vi "sq_test.vi"() -> ()   [LabVIEW 2011]
uses:
  <vilib>/Platform/TimedLoop/XDataNode/timing_clust.ctl
  <vilib>/Platform/TimedLoop/XDataNode/nitl_modes.ctl
  <vilib>/Platform/TimedLoop/XDataNode/wakeup.ctl
  <vilib>/Platform/TimedLoop/XDataNode/XDataNode.xnode
  <vilib>/Platform/TimedLoop/XDataNode/XDNodeRunTimeDep.lvlib
panel:
  in  "Num read":u8
  in  "Init sequences":T1={"Cluster"={"Cmd bytes"=[0, 99, 145], "Send"=FALSE}, "Cluster 2"={"Cmd bytes"=[0, 107, 145, 119, 255], "Send"=FALSE}, "Cluster 3"={"Cmd bytes"=[0, 103, 145, 119, 255], "Send"=FALSE}, "Cluster 4"={"Cmd bytes"=[], "Send"=FALSE}} {"Cluster 4"."Cmd bytes" format="%.0x"; "Cluster 3"."Cmd bytes" format="%.0x"; "Cluster 2"."Cmd bytes" format="%.0x"; "Cluster"."Cmd bytes" format="%.0x"}
  in  "Continuous 2":bool
  in  "Bit rate":dbl=400000.0 min=40000.0 max=2000000.0 format="%#_3p"
  in  "Address":u8=84 max=127 step=1 format="%2x"
  in  "Bus":u8 max=2 step=1
  in  "Pulse count":i16(slide) min=-2047 max=2047 scale=-1700.0..1700.0
  in  "Continuous":bool
  in  "Step":bool
  in  "Send":bool
  in  "stop":bool
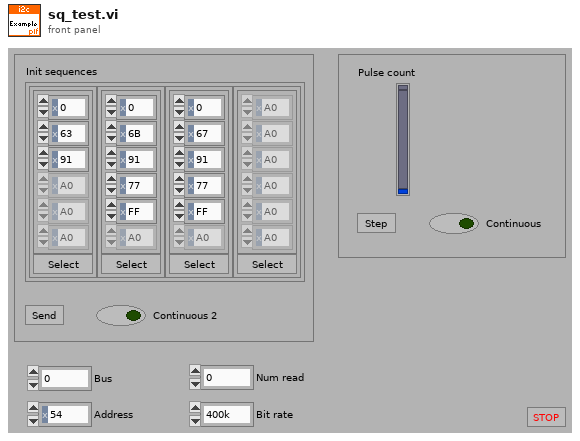
[diagram p1: front panel]
types:
  T1 = cluster{"Cluster":cluster{"Cmd bytes":u8[], "Send":bool}, "Cluster 2":cluster{"Cmd bytes":u8[], "Send":bool}, "Cluster 3":cluster{"Cmd bytes":u8[], "Send":bool}, "Cluster 4":cluster{"Cmd bytes":u8[], "Send":bool}}
  T2 = typedef "i2c_interface.ctl" = cluster{"FPGA VI Reference":T3}
  T3 = typedef "fpga_reference.ctl" = refnum<k20>
  T4 = typedef "XDNodeRunTimeDep.lvlib/timing_clust.ctl" = cluster{"Expected End [f-1]":u64, "Actual End [f-1]":u64, "Finished Late? [f-1]":bool, "Expected End [i-1]":u64, "Actual End [i-1]":u64, "Finished Late? [i-1]":bool, "Expected Start [i]":u64, "Actual Start [i]":u64, "Expected Start [f]":u64, "Actual Start [f]":u64, "Source Name":string, "Structure Name":string, "Period":i64, "Deadline":i64, "Offset":i64, "Start":i64, "Priority":i32, "Timeout":i32, "Mode":T5, "Wakeup Reason":T6, "Error":errorcluster, "Source Type":string, "Secondary Source Type":string, "Global End Time":u64, "Global Start Time":u64, "Frame Duration":u64, "Iteration Duration":u64, "Assigned CPU":i32, "I/O Scan Engine Mode":u32}
  T5 = typedef "XDNodeRunTimeDep.lvlib/nitl_modes.ctl" = enum32{"No Change", "Process missed periods, maintain original phase", "Discard missed periods, maintain original phase", "Process missed periods, ignore original phase", "Discard missed periods, ignore original phase"}
  T6 = typedef "XDNodeRunTimeDep.lvlib/wakeup.ctl" = enum32{"Normal", "Aborted", "Asynchronous wakeup", "Timing source error", "Timed loop error", "Timeout"}
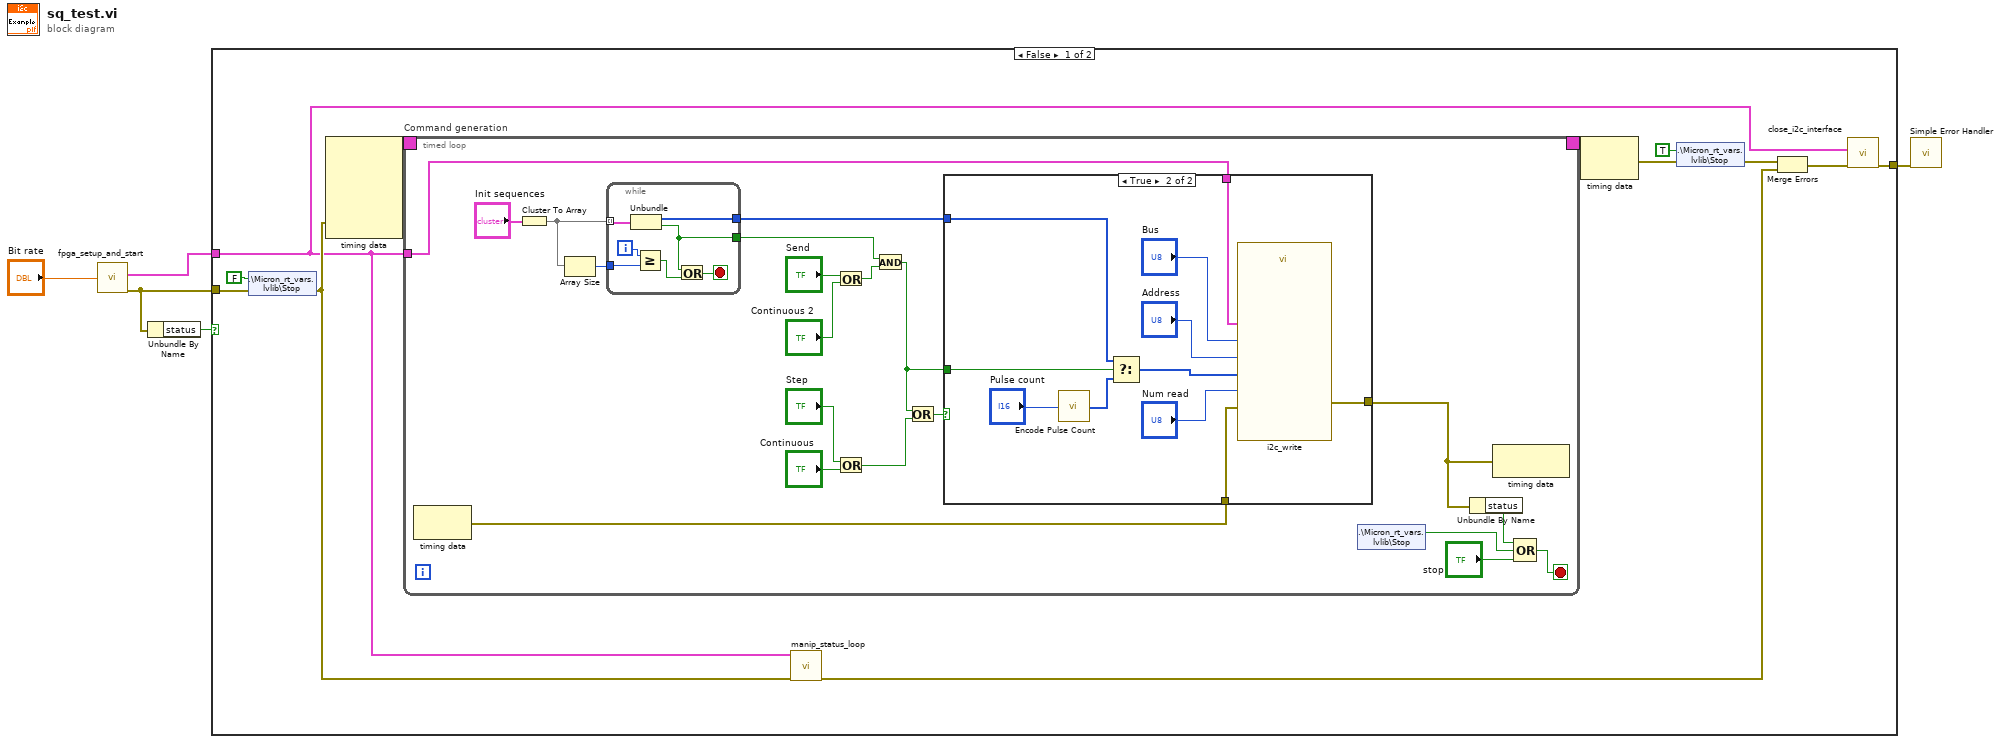
[diagram p0: block diagram]
diagram:
  n1 = call "fpga_setup_and_start.vi"("Bit rate"="Bit rate") -> ("error out"=w3:errorcluster, "I2C interface"=w2:T2)  [unwired: 9 in]
  n2 = Unbundle By Name(w3) -> ("status"=w1:bool)
  n3 = case shown="False" w1 {
    tunnel: [w15 w67] -> w5
    tunnel: w3 -> [w7 w67]
    tunnel: w2 -> [w6 _]
    frame False {
      n4 = shared-variable ".\\Micron_rt_vars.lvlib\\Stop"(FALSE ("Stop"), error in=w7) -> (error out=w8:errorcluster)
      n5 = node-c288(w8) -> (w17:T4)  [unwired: 4 in]
      n6 = timed-loop "Command generation" {
        timing: w17 -> [_]
        timing-out: [_] -> w16
        tunnel: w6 -> [w31]
        stop <- w36 stop-if-true
        n7 = node-c288() -> (w30:errorcluster)  [unwired: 1 in]
        n8 = Cluster To Array(cluster="Init sequences") -> (array=w23:cluster{"Cmd bytes":u8[], "Send":bool}[])
        n9 = Array Size(array=w23) -> (size(s)=w22:i32)
        n10 = while {
          tunnel: w23 -> [w44] mode=indexing
          tunnel: [w43] -> w21
          tunnel: w22 -> [w41]
          tunnel: [w38] -> w19
          i -> [w40]
          stop <- w42 stop-if-true
          n11 = Unbundle(w44) -> ("Cmd bytes"=w43:u8[], "Send"=w38:bool)
          n12 = Greater Or Equal?(x=w40, y=w41) -> (x >= y?=w39:bool)
          n13 = Or(x=w38, y=w39) -> (x .or. y?=w42:bool)
        }
        n14 = Or(x="Send", y="Continuous 2") -> (x .or. y?=w20:bool)
        n15 = Or(x="Step", y="Continuous") -> (x .or. y?=w32:bool)
        n16 = And(x=w19, y=w20) -> (x .and. y?=w18:bool)
        n17 = Or(x=w18, y=w32) -> (x .or. y?=w33:bool)
        n18 = case shown="True" w33 {
          tunnel: w18 -> [_ w56]
          tunnel: w31 -> [_ w53]
          tunnel: w30 -> [w45 w52]
          tunnel: [w45 w51] -> w29
          tunnel: w21 -> [_ w47]
          frame False {
          }
          frame True {
            n19 = call "Encode Pulse Count.vi"("Pulse count"="Pulse count") -> ("Array"=w54:u8[])
            n20 = Select(t=w47, s=w56, f=w54) -> (s? t:f=w50:u8[])
            n21 = call "i2c_write.vi"("Num read"="Num read", "Bus"="Bus", "error in"=w52, "Data"=w50, "Address"="Address", "I2C interface"=w53) -> ("error out"=w51:errorcluster)  [unwired: 4 in, 1 out]
          }
        }
        n22 = shared-variable ".\\Micron_rt_vars.lvlib\\Stop"() -> (w27:bool)  [unwired: 2 out]
        n23 = Unbundle By Name(w29) -> ("status"=w28:bool)
        n24 = node-c288(w29) -> ()  [unwired: 1 out]
        n25 = Compound Arithmetic op=OR(w28, w27, "stop") -> (w36:bool)
      }
      n26 = call "manip_status_loop.vi"("error in"=w8, "I2C interface"=w6) -> ("error out"=w13:errorcluster)  [unwired: 9 in]
      n27 = node-c288(w16) -> (w11:errorcluster)
      n28 = shared-variable ".\\Micron_rt_vars.lvlib\\Stop"(TRUE ("Stop"), error in=w11) -> (error out=w10:errorcluster)
      n29 = Merge Errors(w10, w13) -> (w14:errorcluster)
      n30 = call "close_i2c_interface.vi"("error in"=w14, "I2C interface"=w6) -> ("error out"=w15:errorcluster)  [unwired: 9 in]
    }
    frame True {
    }
  }
  n31 = call <vilib>:"Simple Error Handler.vi"("error in (no error)"=w5) -> ()  [unwired: 4 in, 5 out]
